vi "single move without gyro(VAJ test).vi"(8 "error in (no error)":errorcluster, 9 "RPM":dbl, 10 "Y":dbl, 11 "X":dbl) -> (0 "error out":errorcluster)   [LabVIEW 2019]
uses:
  <vilib>/Platform/TimedLoop/XDataNode/timing_clust.ctl
  <vilib>/Platform/TimedLoop/XDataNode/nitl_modes.ctl
  <vilib>/Platform/TimedLoop/XDataNode/wakeup.ctl
  <vilib>/platform/TimedLoop/XDataNode/XDataNode.xnode
  <vilib>/Platform/TimedLoop/XDataNode/XDNodeRunTimeDep.lvlib
  <vilib>/addons/control/pid/NI_PID_pid.lvlib
  <vilib>/ptbypt/NI_PtbyPt.lvlib
panel:
  in  "V":dbl=75.0
  in  "A":dbl=100.0
  in  "J":dbl=175.0
  out "Waveform Chart":dbl(graph)
  out "out array":dbl[](array[numeric])
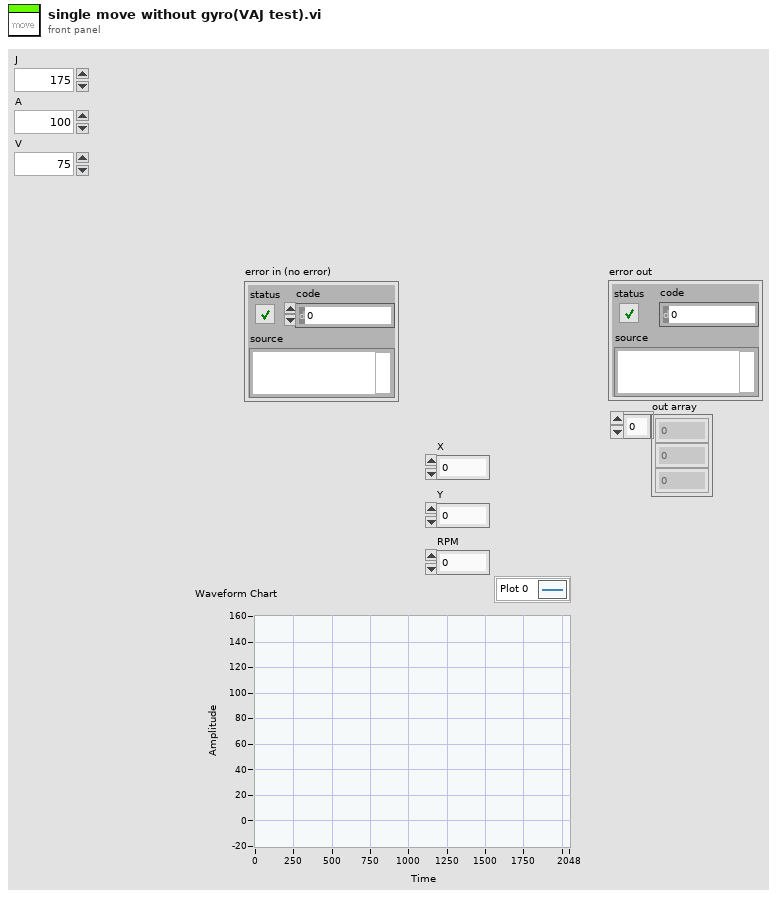
[diagram p1: front panel]
types:
  T1 = typedef "XDNodeRunTimeDep.lvlib/timing_clust.ctl" = cluster{"Expected End [f-1]":u64, "Actual End [f-1]":u64, "Finished Late? [f-1]":bool, "Expected End [i-1]":u64, "Actual End [i-1]":u64, "Finished Late? [i-1]":bool, "Expected Start [i]":u64, "Actual Start [i]":u64, "Expected Start [f]":u64, "Actual Start [f]":u64, "Source Name":string, "Structure Name":string, "Period":i64, "Deadline":i64, "Offset":i64, "Start":i64, "Priority":i32, "Timeout":i32, "Mode":T2, "Wakeup Reason":T3, "Error":errorcluster, "Source Type":string, "Secondary Source Type":string, "Global End Time":u64, "Global Start Time":u64, "Frame Duration":u64, "Iteration Duration":u64, "Assigned CPU":i32, "I/O Scan Engine Mode":u32}
  T2 = typedef "XDNodeRunTimeDep.lvlib/nitl_modes.ctl" = enum32{"No Change", "Process missed periods, maintain original phase", "Discard missed periods, maintain original phase", "Process missed periods, ignore original phase", "Discard missed periods, ignore original phase"}
  T3 = typedef "XDNodeRunTimeDep.lvlib/wakeup.ctl" = enum32{"Normal", "Aborted", "Asynchronous wakeup", "Timing source error", "Timed loop error", "Timeout"}
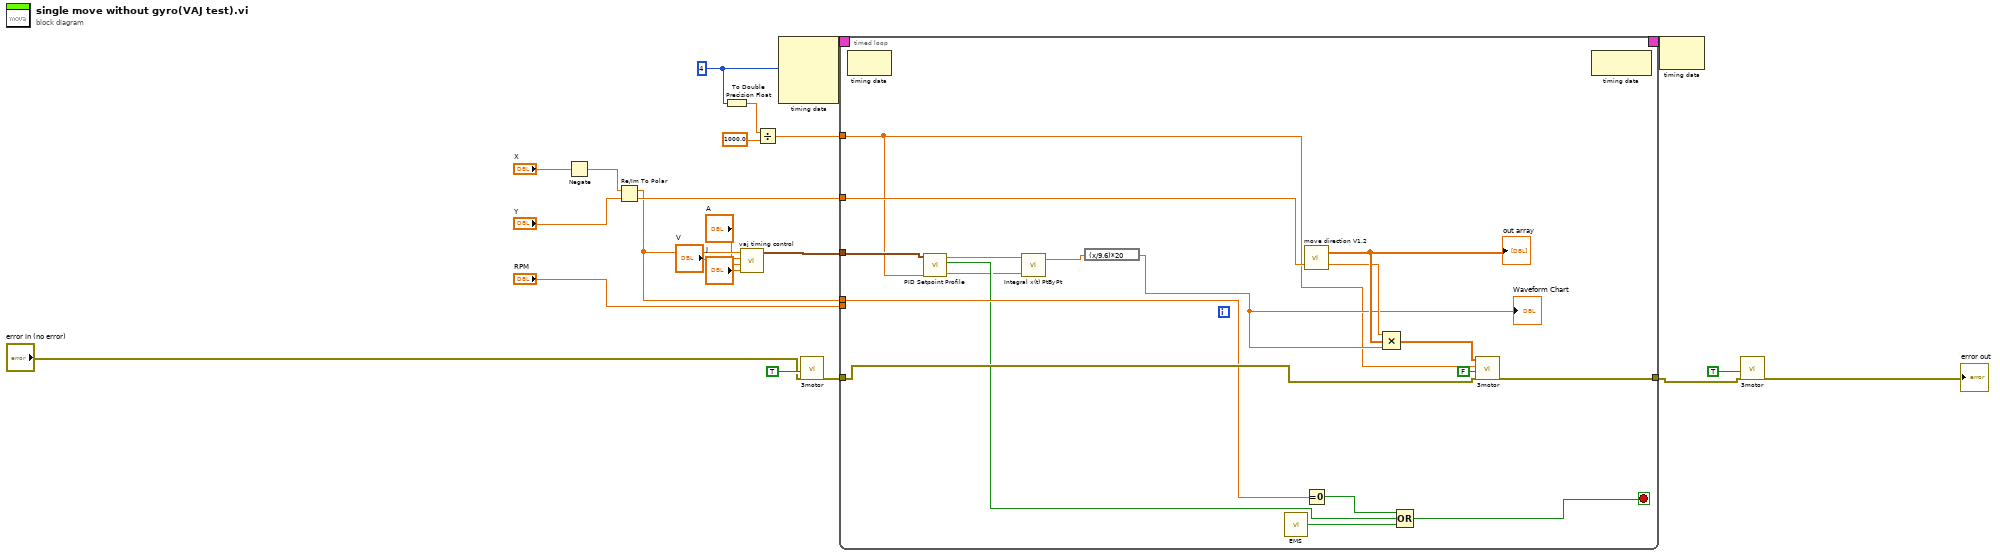
[diagram p0: block diagram]
diagram:
  w20 = i64 4 ("Period")
  n1 = Negate(x="X") -> (-x=w8:dbl)
  n2 = Re/Im To Polar(2:"Y", 3:w8) -> (0:w15:dbl, 1:w5:dbl)
  n3 = To Double Precision Float(number=w20) -> (double precision float=w19:dbl)
  n4 = call "vaj timing control.vi"("J"="J", "A"="A", "V"="V", "D"=w5) -> ("Array"=w4:cluster{"Numeric":dbl, "Numeric":dbl}[])  [unwired: 7 in]
  n5 = Divide(x=w19, y=1000.0) -> (x/y=w17:dbl)
  n6 = node-c288(w20) -> (w22:T1)  [unwired: 3 in]
  n7 = call "3motor.vi"("error in (no error)"="error in (no error)", "Reset"=TRUE) -> ("error out"=w13:errorcluster)  [unwired: 8 in, 1 out]
  n8 = timed-loop {
    timing: w22 -> [_]
    timing-out: [_] -> w21
    tunnel: w17 -> [w23]
    tunnel: w15 -> [w40]
    tunnel: w5 -> [w31]
    tunnel: "RPM" -> [_]
    tunnel: w13 -> [w35]
    tunnel: [w39] -> w7
    tunnel: w4 -> [w29]
    stop <- w37 stop-if-true
    n9 = node-c288() -> ()  [unwired: 1 in, 1 out]
    n10 = call <vilib>:"PID Setpoint Profile.vi"("dt (s)"=w23, "setpoint profile"=w29) -> ("dt out (s)"=w26:dbl, "profile complete?"=w28:bool, "setpoint"=w27:dbl)  [unwired: 4 in, 1 out]
    n11 = call <vilib>:"Integral x(t) PtByPt.vi"("dt"=w26, "x"=w27) -> ("integral x(t)"=w25:dbl)  [unwired: 2 in, 1 out]
    n12 = expression code="(x/9.6)*20"(w25) -> (w24:dbl)
    "Waveform Chart" <- w24
    n13 = call "EMS.vi"() -> ("A/DIO4 (Pin 19)"=w34:bool)
    n14 = call "move direction V1.2.vi"("theta"=w40) -> ("max value"=w30:dbl, "out array"=w32:dbl[])  [unwired: 1 in]
    "out array" <- w32
    n15 = Equal To 0?(x=w31) -> (x = 0?=w36:bool)
    n16 = Compound Arithmetic op=MULTIPLY(w30, w32, w24) -> (w38:dbl[])
    n17 = Compound Arithmetic op=OR(w36, w28, w34) -> (w37:bool)
    n18 = call "3motor.vi"("error in (no error)"=w35, "Reset"=FALSE, "dt(s)"=w23, "Motor speed"=w38) -> ("error out"=w39:errorcluster)  [unwired: 6 in, 1 out]
    n19 = node-c288() -> ()  [unwired: 1 in, 1 out]
  }
  n20 = node-c288(w21) -> ()  [unwired: 1 out]
  n21 = call "3motor.vi"("error in (no error)"=w7, "Reset"=TRUE) -> ("error out"=→"error out":errorcluster)  [unwired: 8 in, 1 out]
